vi "Do Attacks.vi"(6 "Teams in":refnum<class "Team.lvclass">[](array[class]), 9 "New Map in":refnum<class "Map.lvclass">) -> (1 "New Map out":refnum<class "Map.lvclass">, 4 "Teams out":refnum<class "Team.lvclass">[](array[class]))   [LabVIEW 2020, in "SquareBattle.lvlib" / "Map.lvclass"]
uses:
  Map.lvclass
  Team/Team.lvclass
  Map.lvclass/Map.ctl
  Square/Square.lvclass
  Team/Team.lvclass/Team.ctl
  Team Stats.ctl
  SquareBattle.lvlib
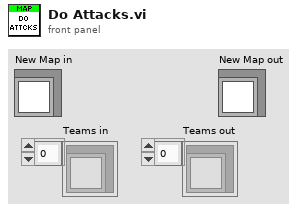
[diagram p1: front panel]
types:
  T1 = typedef "SquareBattle.lvlib/Team Stats.ctl" = cluster{"Active":i32, "Generated":i32, "Kills":i32, "Eliminated":i32, "Collided":i32}
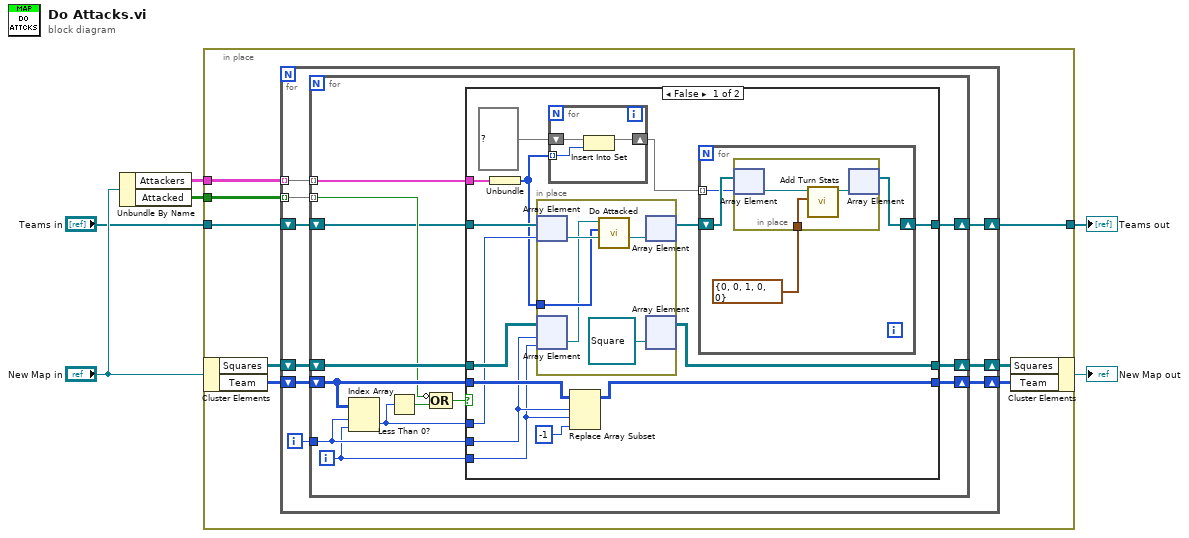
[diagram p0: block diagram]
diagram:
  n1 = Unbundle By Name("New Map in") -> ("Attackers"=w1:cluster{"Array":i32[]}[][], "Attacked"=w5:bool[][])
  n2 = in-place {
    in-place-border: w5 -> [w12]
    in-place-border: "Teams in" -> [w11]
    in-place-border: [w10] -> w3
    in-place-border: w1 -> [w7]
    n3 = in-place-cluster #1("New Map in") -> ("Squares"=w14:refnum<class "Square.lvclass">[][], "Team"=w13:i32[][])
    n4 = for {
      shift-right: [w17] -> w8
      shift-left: w13 -> [w22]
      shift-right: [w18] -> w9
      shift-left: w14 -> [w23]
      tunnel: w12 -> [w21] mode=indexing
      shift-right: [w16] -> w10
      shift-left: w11 -> [w20]
      tunnel: w7 -> [w15] mode=indexing
      i -> [w19]
      n5 = for {
        shift-right: [w29] -> w18
        shift-left: w23 -> [w35]
        shift-right: [w30] -> w17
        shift-left: w22 -> [w36]
        tunnel: w21 -> [w32] mode=indexing
        shift-right: [w27] -> w16
        shift-left: w20 -> [w28]
        tunnel: w19 -> [w26]
        tunnel: w15 -> [w24] mode=indexing
        i -> [w25]
        n6 = Index Array(array=w36, index (row)=w26, index (col)=w25) -> (element=w34:i32)
        n7 = Less Than 0?(x=w34) -> (x < 0?=w33:bool)
        n8 = Compound Arithmetic op=OR(invert w32, w33) -> (w31:bool)
        n9 = case shown="False" w31 {
          tunnel: w36 -> [w47 w69]
          tunnel: w35 -> [w49 w68]
          tunnel: w34 -> [w42 _]
          tunnel: [w46 w69] -> w30
          tunnel: [w48 w68] -> w29
          tunnel: w28 -> [w50 w67]
          tunnel: [w38 w67] -> w27
          tunnel: w26 -> [w45 _]
          tunnel: w25 -> [w44 _]
          tunnel: w24 -> [w51 _]
          frame False {
            n10 = Unbundle(w51) -> ("Array"=w41:i32[])
            n11 = in-place {
              in-place-border: w41 -> [w64]
              n12 = in-place-array #2(w50, w42) -> (w65:refnum<class "Team.lvclass">)
              n13 = in-place-array #3(w49, w45, w44) -> (w63:refnum<class "Square.lvclass">)
              n14 = call "Do Attacked.vi"("Team In"=w65, "Attackers"=w64, "Square"=w63) -> ("Team out"=w62:refnum<class "Team.lvclass">)  [unwired: 8 in]
              n15 = in-place-array #2(w62) -> (w39:refnum<class "Team.lvclass">[])  [unwired: 1 out]
              n16 = in-place-array #3(refnum<class "Square.lvclass"> refnum ("element")) -> (w48:refnum<class "Square.lvclass">[][])  [unwired: 2 out]
            }
            n17 = for {
              tunnel: w41 -> [w61] mode=indexing
              shift-right: [w59] -> w37
              shift-left: set{i32} {} ("set in") -> [w60]
              n18 = Insert Into Set(10:w61, 11:w60) -> (3:w59:set{i32})  [unwired: 1 out]
            }
            n19 = Replace Array Subset(array=w47, new element=-1 ("new element/subarray"), index (row)=w45, index (col)=w44) -> (w46:i32[][])
            n20 = for {
              shift-right: [w52] -> w38
              shift-left: w39 -> [w54]
              tunnel: w37 -> [w53] mode=indexing
              n21 = in-place {
                in-place-border: T1 {"Active"=0, "Generated"=0, "Kills"=1, "Eliminated"=0, "Collided"=0} ("Team Stats") -> [w58]
                n22 = in-place-array #4(w54, w53) -> (w57:refnum<class "Team.lvclass">)
                n23 = call "Add Turn Stats.vi"("Team Stats"=w58, "Team in"=w57) -> ("Team out"=w56:refnum<class "Team.lvclass">)  [unwired: 9 in]
                n24 = in-place-array #4(w56) -> (w52:refnum<class "Team.lvclass">[])  [unwired: 1 out]
              }
            }
          }
          frame True {
            # "Not being attacked or empty, do nothing."
          }
        }
      }
    }
    n25 = in-place-cluster #1("Squares"=w9, "Team"=w8) -> (→"New Map out":refnum<class "Map.lvclass">)
  }
  "Teams out" <- w3
